vi "Query Event Log Last Entries.vi"(8 "error in (no error)":errorcluster, 10 "Count (1)":i32=1, 11 "VISA resource name":refnum<visa-resource-name>) -> (0 "error out":errorcluster, 3 "VISA resource name out":refnum<visa-resource-name>)   [LabVIEW 2020, in "Rohde&Schwarz CMXP Base.lvlib"]
doc: "Queries the specified number entries of the event log.\n\nAttribute:\nRSCMXPBASE_ATTR_EVENT_LOG_LAST_ENTRIES\n\nRemote-control command:\nSENSe:ELOG:LAST?"
uses:
  <instrlib>/Rohde&Schwarz CMXP Base/Rohde&Schwarz CMXP Base.lvlib
  <instrlib>/Rohde&Schwarz CMXP Base/Private/rsidr_core.llb/rsidr_core.lvlib
panel:
  out "Event Logs":T1(array[cluster])
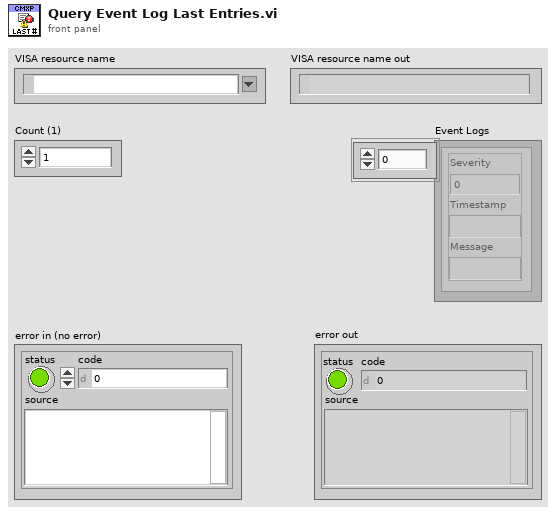
[diagram p1: front panel]
types:
  T1 = cluster{"Severity":dbl, "Timestamp":string, "Message":string}[]
  T2 = cluster{"Severity":i32, "Timestamp":string, "Message":string}
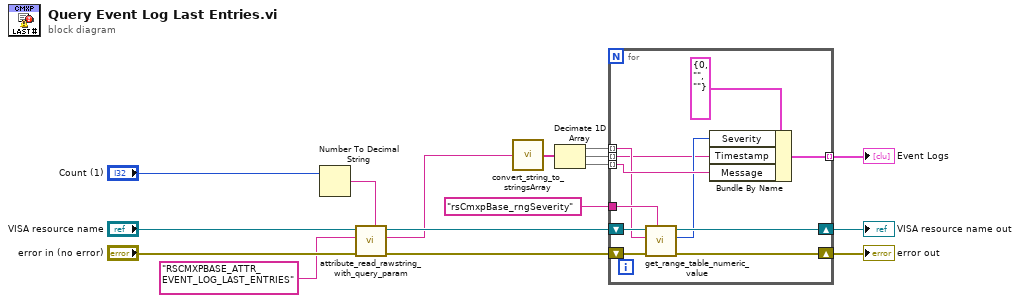
[diagram p0: block diagram]
diagram:
  n1 = Number To Decimal String(number="Count (1)") -> (decimal integer string=w4:string)  [unwired: 1 in]
  n2 = call <instrlib>:"attribute_read_rawstring_with_query_param.vi"("Query Parameter (None)"=w4, "error in"="error in (no error)", "Attribute ID"="RSCMXPBASE_ATTR_EVENT_LOG_LAST_ENTRIES", "VISA resource name"="VISA resource name") -> ("error out"=w2:errorcluster, "RawString out"=w1:string, "VISA resource name out"=w3:refnum<visa-resource-name>)  [unwired: 5 in]
  n3 = call <instrlib>:"convert_string_to_stringsArray.vi"("String in"=w1) -> ("string array out"=w16:string[])  [unwired: 3 in, 1 out]
  n4 = Decimate 1D Array(w16) -> (w15:string[], w14:string[], w13:string[])
  n5 = for {
    tunnel: w15 -> [w19] mode=indexing
    tunnel: w14 -> [w17] mode=indexing
    tunnel: w13 -> [w26] mode=indexing
    tunnel: [w25] -> w9 mode=indexing
    tunnel: "rsCmxpBase_rngSeverity" ("Range Table ID in") -> [w24]
    shift-right: [w20] -> w11
    shift-left: w3 -> [w23]
    shift-right: [w21] -> w10
    shift-left: w2 -> [w22]
    n6 = call <instrlib>:"get_range_table_numeric_value.vi"("Range Table ID in"=w24, "error in"=w22, "String Value"=w19, "VISA resource name"=w23) -> ("error out"=w21:errorcluster, "I32 output"=w18:i32, "VISA resource name out"=w20:refnum<visa-resource-name>)  [unwired: 5 in]
    n7 = Bundle By Name(cluster=T2 {"Severity"=0, "Timestamp"="", "Message"=""} ("Event Logs 2"), "Severity"=w18, "Timestamp"=w17, "Message"=w26) -> (w25:T2)
  }
  "error out" <- w10
  "VISA resource name out" <- w11
  "Event Logs" <- w9
